vi "Car Moved Out of Position.vi"(8 "error in (no error)":errorcluster, 11 "Simulated Wash Display Console in":refnum<class "Simulated Wash Display Console.lvclass">) -> (0 "error out":errorcluster, 3 "Simulated Wash Display Console out":refnum<class "Simulated Wash Display Console.lvclass">)   [LabVIEW 2012, in "Simulated Wash Display Console.lvlib" / "Simulated Wash Display Console.lvclass"]
uses:
  Simulated Wash Display Console.lvclass
  Wash Display Console API/Wash Display Console API/Wash Display Console API.lvclass
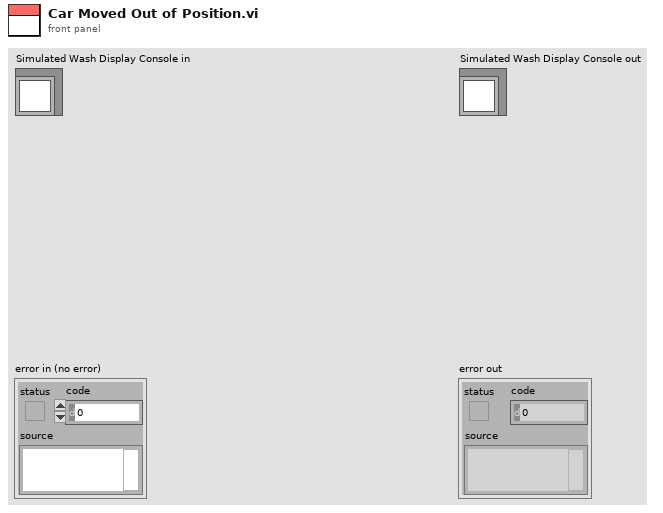
[diagram p1: front panel]
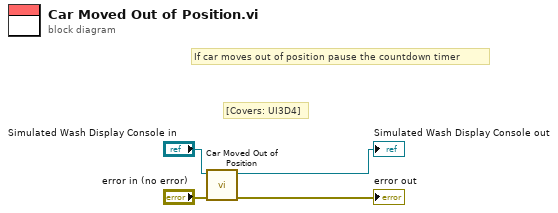
[diagram p0: block diagram]
diagram:
  # "[Covers: UI3D4]"
  # "If car moves out of position pause the countdown timer"
  n1 = call-parent "Car Moved Out of Position.vi"("error in (no error)"="error in (no error)", "Wash Display Console API in"="Simulated Wash Display Console in") -> ("error out"=→"error out":errorcluster, "Wash Display Console API out"=→"Simulated Wash Display Console out":refnum<class "Simulated Wash Display Console.lvclass">)  [unwired: 8 in]
